vi "Perform AC Measurements.vi"(5 "stop frequency":dbl, 7 "start frequency":dbl, 8 "error in (no error)":errorcluster, 9 "analog waveform":waveform(dbl), 10 "input range (pk)":dbl=1.0 format="%^.1e") -> (0 "error out":errorcluster, 2 "AC measurement results":T1, 3 "frequency domain":cluster{"x0":dbl, "dx":dbl, "magnitude":dbl[]} {"magnitude" format="%.2p"; "dx" format="%.2p"; "x0" format="%.2p"})   [LabVIEW 2021, in "adc_acMultiChannelMeasurement.lvlib"]
uses:
  <vilib>/addons/_NISVFA/_Shared subVIs/Controls/svc_Window.ctl
  <vilib>/addons/_NISVFA/_Shared subVIs/Common/SVL Set dB Reference (1 Ch).vi
  <vilib>/addons/_NISVFA/_Spectrum Processing/SVFA Get Spectrum Subset (Complex) (1 Ch).vi
  <vilib>/addons/_NISVFA/_Spectrum Processing/SVFA Unit Conversion (Complex) (1 Ch).vi
  <vilib>/addons/_NISVFA/_Shared subVIs/Common/SVL Set dB Reference (variant).vi
  <vilib>/addons/_NISVFA/_Shared subVIs/Common/svc_Check Frequency Range in Spectrum.vi
  <vilib>/addons/_NISVFA/_Shared subVIs/Common/svc_Build Unit Label for Frequency Range.vi
  <vilib>/addons/_NISVFA/_Shared subVIs/Common/svc_Window Parameters.vi
  <vilib>/addons/_NISVFA/_Shared subVIs/Common/svc_Extract Single Tone Information (complex).vi
  <vilib>/addons/_NISVFA/_Spectrum Processing/SVFA Spectrum Peak Search.vi
  <vilib>/addons/_NISVFA/_Spectrum Processing/SVFA Spectrum Peak Search (1 Ch).vi
  <vilib>/addons/_NISVFA/_Shared subVIs/Common/svc_Spectrum Units.vi
  <vilib>/addons/_NISVFA/_Shared subVIs/Common/svc_Log View for Spectrum (1Ch).vi
  <vilib>/addons/_NISVFA/_Spectrum Processing/SVFA Unit Conversion (1 Ch).vi
  <vilib>/addons/_NISVFA/_Shared subVIs/Common/svc_Complex Datatype Defaults.vi
  <vilib>/addons/_NISVFA/_Shared subVIs/Common/svc_Check Frequency Range in Bandwidth.vi
  <vilib>/addons/_NISVFA/_Shared subVIs/Common/svc_Convert Start and Stop to Start Index and Length.vi
  <vilib>/addons/_NISVFA/_Spectrum Processing/SVFA Get Tone Amplitude and Phase (1 Ch).vi
  <vilib>/addons/_NISVFA/_Spectrum Processing/subVIs/svfa_Compute Complex Spectrum for Export.vi
  <vilib>/addons/_NISVFA/_Spectrum Processing/subVIs/svfa_Spectrum Peak Search.vi
  <vilib>/addons/_NISVFA/_Shared subVIs/Common/svc_Format Value (DBL).vi
  <vilib>/addons/_NISVFA/_Shared subVIs/Common/svc_Get Weighting Enum and Labels.vi
  <vilib>/addons/_NISVFA/_Shared subVIs/Common/svc_Engineering Units to Unit Label.vi
  <vilib>/addons/_NISVFA/_Shared subVIs/Common/svc_Surround NonAlpha String with Parentheses.vi
  <vilib>/dlg_ctls.llb/Space Constant.vi
  <vilib>/addons/_NISVFA/_Shared subVIs/Common/svc_Unwrap Phase.vi
  <vilib>/addons/_NISVFA/_Shared subVIs/Common/svc_Convert Spectrum Array to dB.vi
  <vilib>/addons/_NISVFA/_Spectrum Processing/subVIs/svfa_Conversion Utility (spectrum info).vi
  <vilib>/addons/_NISVFA/_Spectrum Processing/subVIs/svfa_Window Frequency Response.vi
  <vilib>/addons/_NISVFA/_Spectrum Processing/subVIs/svfa_Window Frequency Response (double array).vi
  <vilib>/Analysis/baseanly.llb/Dot Product.vi
  <vilib>/Analysis/baseanly.llb/Complex Dot Product.vi
  <vilib>/addons/_NISVFA/_Spectrum Processing/subVIs/svfa_Peak Rough Search Indices.vi
  <vilib>/addons/_NISVFA/_Shared subVIs/Common/svc_Unit Label Lexical Class.vi
  <vilib>/addons/_NISVFA/_Spectrum Processing/subVIs/svfa_Peak to RMS to Peak2Peak.vi
  <vilib>/addons/_NISVFA/_Spectrum Processing/subVIs/svfa_Mag to Mag2.vi
  <vilib>/addons/_NISVFA/_Spectrum Processing/subVIs/svfa_Linear to dB.vi
  <vilib>/addons/_NISVFA/_Spectrum Processing/subVIs/svfa_dBrefA to dBrefB.vi
  <vilib>/addons/_NISVFA/_Spectrum Processing/subVIs/svfa_Spectrum to Spectral Density.vi
  <vilib>/addons/_NISVFA/_Spectrum Processing/subVIs/svfa_Rect Window Frequency Response.vi
  <vilib>/addons/_NISVFA/_Spectrum Processing/subVIs/svfa_Cosine Window Coefficients.vi
  <vilib>/addons/_NISVFA/_Shared subVIs/Common/svc_Caller VI Returned in Error Source.vi
  <vilib>/addons/_NISVFA/_Baseband FFT/SVFA FFT Spectrum (Complex) (1 Ch).vi
  <vilib>/addons/_NISVFA/_Shared subVIs/Common/svc_Convert Frequency to Frequency String.vi
  <vilib>/addons/Sound and Vibration/svt_Single Tone Measurements/SVT Gain (Frequency) (1 Ch).vi
  <vilib>/Analysis/4window.llb/window parameters.vi
  <vilib>/Analysis/4window.llb/Window Properties.vi
  <vilib>/Analysis/4window.llb/Window Properties by Name.vi
  <vilib>/addons/_NISVFA/_Spectrum Processing/subVIs/svfa_Spectrum Peak Tone Search and Estimation (complex).vi
  <vilib>/measure/masignal.llb/Tones and Noise Waveform.vi
  <vilib>/addons/_NISVFA/_Shared subVIs/Common/svc_FFT with Window.vi
  <vilib>/Analysis/1siggen.llb/Square Wave.vi
  <vilib>/addons/_NISVFA/_Spectrum Processing/subVIs/svfa_Three Finger Peak Search.vi
  <vilib>/addons/Sound and Vibration/svt_Distortion/subVIs/sv_Peak View Amplitude (1 Ch).vi
  adc_acMultiChannelMeasurement.lvlib
  <vilib>/addons/Sound and Vibration/svt_Distortion/SoundVib_Distortion.lvlib
  <vilib>/addons/Sound and Vibration/svt_Single Tone Measurements/SoundVib_SingleTone.lvlib
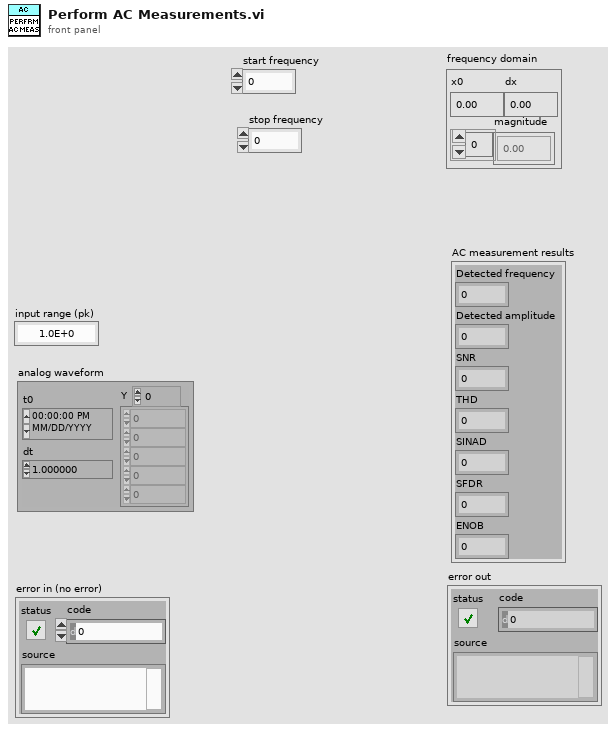
[diagram p1: front panel]
types:
  T1 = cluster{"Detected frequency":dbl, "Detected amplitude":dbl, "SNR":dbl, "THD":dbl, "SINAD":dbl, "SFDR":dbl, "ENOB":dbl}
  T2 = enum16{"no change", "spectrum", "spectral density"}
  T3 = cluster{"linear/dB":enum16{"no change", "linear", "dB"}, "dB reference (0: no change)":dbl, "power/magnitude":enum16{"no change", "power", "magnitude"}, "view":enum16{"no change", "rms", "peak", "peak-peak"}}
  T4 = typedef "svc_Window.ctl" = u32
  T5 = typedef "svc_Spectrum Info.ctl" = cluster{"channel name":string, "description":string, "x-axis units":T6, "spectral info":cluster{"spectrum type":T7, "linear/dB":enum16{"linear", "dB"}, "window":u16, "window size":i32, "FFT size":i32}, "engineering units":T8, "custom label":string, "dB reference [EU]":dbl, "peak units":enum16{"rms", "peak", "peak-peak"}, "weighting filter":T9, "spectral density?":bool, "unit label":string, "spectrum skewed?":bool, "complimentary spectrum units":T10}
  T6 = typedef "svc_X-Axis Units.ctl" = u16
  T7 = typedef "svc_Spectrum Type.ctl" = enum16{"FFT Spectrum [complex]", "Amplitude [Magnitude]", "Power [Magnitude^2]", "Cross Spectrum [complex]", "Frequency Response [Complex]"}
  T8 = typedef "svc_Engineering Units Text Ring.ctl" = u16
  T9 = typedef "svc_Weighting Filter Text Ring.ctl" = u16
  T10 = typedef "svc_Complimentary Spectrum Units.ctl" = enum16{"none", "radians", "degrees", "cycles", "imaginary"}
  T11 = cluster{"complex spectrum response":cluster{"f0":dbl, "df":dbl, "complex spectrum":cdb[]}, "spectrum info":T5}
  T12 = cluster{"complex spectrum subset":cluster{"x0":dbl, "dx":dbl, "complex array":cdb[]}, "spectrum info":T5}
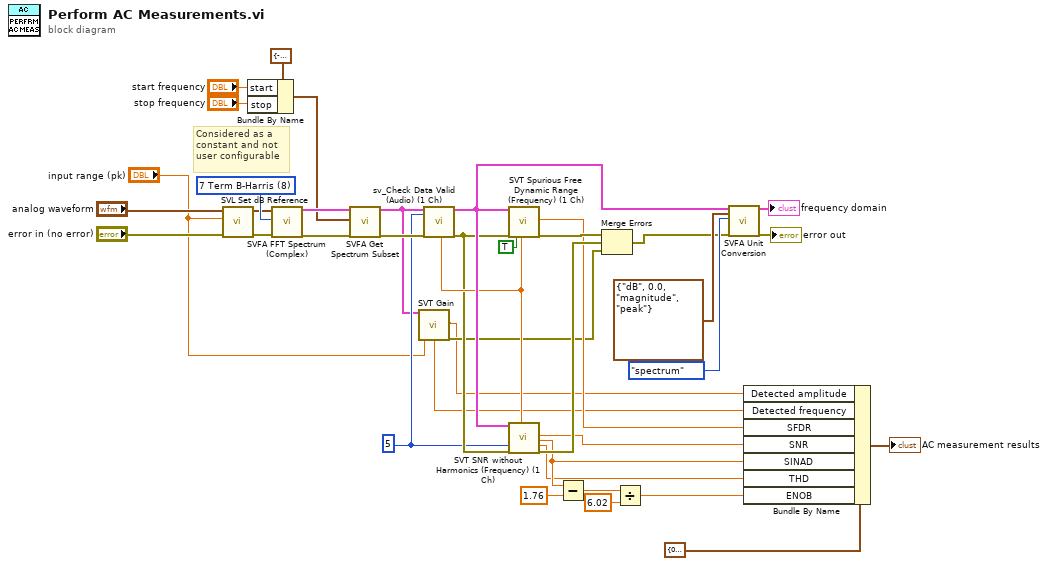
[diagram p0: block diagram]
diagram:
  w18 = 5 ("ACMeasNumberofHarmonics")
  w36 = T4 8 items=["None ", "Hanning", "Hamming", "Blackman-Harris", "Exact Blackman", "Blackman", "Flat Top", "4 Term B-Harris ", "7 Term B-Harris", "Low Sidelobe"] ("window")
  # "Considered as a \nconstant and not\nuser configurable"
  n1 = call-poly <vilib>:"SVL Set dB Reference.vi"("error in (no error)"="error in (no error)", "dB reference [EU]"="input range (pk)", "scaled signal in [EU]"="analog waveform") -> ("error out"=w37:errorcluster, "scaled signal out [EU]"=w33:waveform(dbl))  [unwired: 7 in]
  n2 = Bundle By Name(cluster=cluster{"start":dbl, "stop":dbl} {"start"=-1.0, "stop"=-1.0} ("range"), "start"="start frequency", "stop"="stop frequency") -> (w27:cluster{"start":dbl, "stop":dbl})
  n3 = call-poly <vilib>:"SVFA FFT Spectrum (Complex).vi"("scaled signal [EU]"=w33, "window"=w36, "error in"=w37) -> ("complex spectrum"=w32:T11, "error out"=w31:errorcluster)  [unwired: 13 in, 2 out]
  n4 = call-poly <vilib>:"SVFA Get Spectrum Subset.vi"("complex spectrum"=w32, "range"=w27, "error in (no error)"=w31) -> ("complex spectrum subset"=w5:T12, "error out"=w25:errorcluster)  [unwired: 13 in, 2 out]
  n5 = call-poly <vilib>:"SVT Gain.vi"("complex spectrum"=w5, "amplitude [EU peak]"="input range (pk)") -> ("detected fundamental\nfrequency [Hz]"=w3:dbl, "gain"=w1:dbl, "error out"=w2:errorcluster)  [unwired: 12 in, 3 out]
  n6 = call <vilib>:"sv_Check Data Valid (Audio) (1 Ch).vi"("complex spectrum"=w5, "error in (no error)"=w25, "maximum harmonic"=w18) -> ("dup expected fundamental frequency [Hz]"=w24:dbl, "complex spectrum"=w26:T11, "error out"=w22:errorcluster)  [unwired: 9 in, 5 out]
  n7 = call <vilib>:"SVT Spurious Free Dynamic Range (Frequency) (1 Ch).vi"("complex spectrum"=w26, "error in (no error)"=w22, "exclude harmonics"=TRUE, "expected fundamental\nfrequency [Hz]"=w24) -> ("spurious free dynamic range"=w14:dbl, "error out"=w20:errorcluster)  [unwired: 8 in, 6 out]
  n8 = call <vilib>:"SVT SNR without Harmonics (Frequency) (1 Ch).vi"("complex spectrum"=w26, "maximum harmonic"=w18, "error in (no error)"=w22, "expected fundamental frequency [Hz]"=w24) -> ("SNR (without harmonics)"=w11:dbl, "SINAD"=w10:dbl, "THD"=w9:dbl, "error out"=w21:errorcluster)  [unwired: 8 in, 4 out]
  n9 = Subtract(x=w10, y=1.76) -> (x-y=w7:dbl)
  n10 = Merge Errors(w20, w21, w2) -> (w19:errorcluster)
  n11 = Divide(x=w7, y=6.02) -> (x/y=w15:dbl)
  n12 = call-poly <vilib>:"SVFA Unit Conversion.vi"("complex spectrum"=w26, "desired scaling"=T3 {"linear/dB"=enum."dB", "dB reference (0: no change)"=0.0, "power/magnitude"=enum."magnitude", "view"=enum."peak"}, "spectral density desired"=T2."spectrum", "error in (no error)"=w19) -> ("converted spectrum"=→"frequency domain":cluster{"x0":dbl, "dx":dbl, "magnitude":dbl[]}, "error out"=→"error out":errorcluster)  [unwired: 10 in, 4 out]
  n13 = Bundle By Name(cluster=T1 {"Detected frequency"=0.0, "Detected amplitude"=0.0, "SNR"=0.0, "THD"=0.0, "SINAD"=0.0, "SFDR"=0.0, "ENOB"=0.0} ("AC Measurement Results"), "Detected amplitude"=w1, "Detected frequency"=w3, "SFDR"=w14, "SNR"=w11, "SINAD"=w10, "THD"=w9, "ENOB"=w15) -> (→"AC measurement results":T1)
